vi "Run_VI.vi"(8 "Nome.vi":string, 11 "Origem_VI":enum16{"VI_esta_no_meu_PC", "VI_esta_na_rede"}(ring)) -> (0 "error out":errorcluster, 3 "reference out":refnum<vi>)   [LabVIEW 2019]
panel:
  out "appended path":path
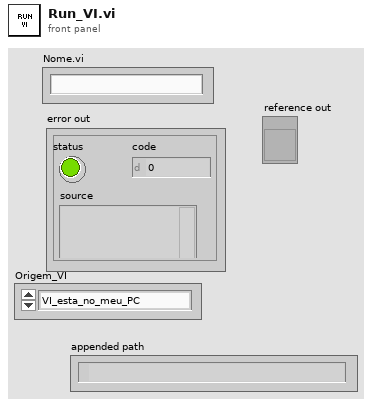
[diagram p1: front panel]
types:
  T1 = enum32{"Bad", "Idle", "Run top level", "Running"}
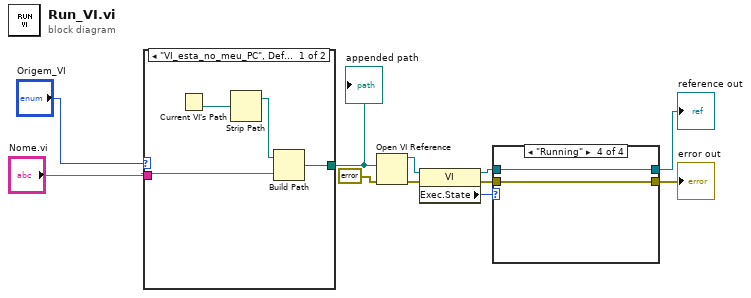
[diagram p0: block diagram]
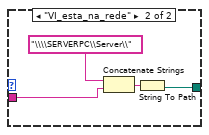
[diagram p2: hidden frame]
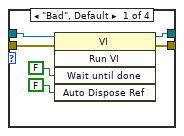
[diagram p3: hidden frame]
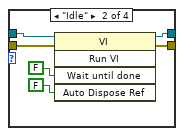
[diagram p4: hidden frame]
diagram:
  n1 = case shown="\"VI_esta_no_meu_PC\", Default" "Origem_VI" {
    tunnel: [w13 w16] -> w10
    tunnel: "Nome.vi" -> [w12 w18]
    frame "VI_esta_no_meu_PC", Default {
      n2 = Current VI's Path() -> (path=w15:path)
      n3 = Strip Path(path=w15) -> (stripped path=w14:path)  [unwired: 1 out]
      n4 = Build Path(base path=w14, name or relative path=w12) -> (appended path=w13:path)
    }
    frame "VI_esta_na_rede" {
      n5 = Concatenate Strings("\\\\SERVERPC\\Server\\", w18) -> (w17:string)
      n6 = String To Path(string=w17) -> (path=w16:path)
    }
  }
  "appended path" <- w10
  n7 = Open VI Reference(vi path=w10, error in (no error)=errorcluster {"status"=FALSE, "code"=0, "source"=""}) -> (vi reference=w7:refnum<vi>, error out=w6:errorcluster)  [unwired: 4 in]
  n8 = property class="VI"(reference=w7, error in=w6) -> (reference out=w4:refnum<vi>, error out=w3:errorcluster, "Exec.State"=w5:T1)
  n9 = case shown="\"Running\"" w5 {
    tunnel: [w23 w29 w33 w35] -> w8
    tunnel: [w22 w28 w32 w34] -> w2
    tunnel: w4 -> [w21 w27 w33 w35]
    tunnel: w3 -> [w20 w26 w32 w34]
    frame "Bad", Default {
      n10 = invoke class="VI" method="Run VI"(reference=w21, error in=w20, "Wait until done"=FALSE ("Wait Until Done"), "Auto Dispose Ref"=FALSE ("Auto Dispose Reference")) -> (reference out=w23:refnum<vi>, error out=w22:errorcluster)  [unwired: 1 in, 3 out]
    }
    frame "Idle" {
      n11 = invoke class="VI" method="Run VI"(reference=w27, error in=w26, "Wait until done"=FALSE ("Wait Until Done"), "Auto Dispose Ref"=FALSE ("Auto Dispose Reference")) -> (reference out=w29:refnum<vi>, error out=w28:errorcluster)  [unwired: 1 in, 3 out]
    }
    frame "Run top level" {
    }
    frame "Running" {
    }
  }
  "reference out" <- w8
  "error out" <- w2
